vi "SearchTemplates.vi"(10 "Search Text":string, 11 "Filtered Templates":refnum<class "MetaDataObj.lvclass">[](array[class])) -> (3 "Display Templates":refnum<class "MetaDataObj.lvclass">[](array[class]))   [LabVIEW 2016]
uses:
  <resource>/dialog/NewProjectWizard/MetaDataObj/MetaDataObj.lvclass
  <resource>/dialog/NewProjectWizard/MetaDataObj/Accessors/Read Title.vi
  <resource>/dialog/NewProjectWizard/MetaDataObj/Accessors/Read Keywords.vi
  <resource>/dialog/NewProjectWizard/MetaDataObj/Accessors/Read Description.vi
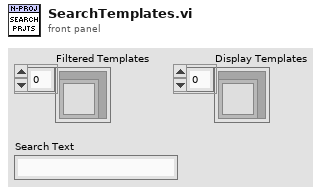
[diagram p1: front panel]
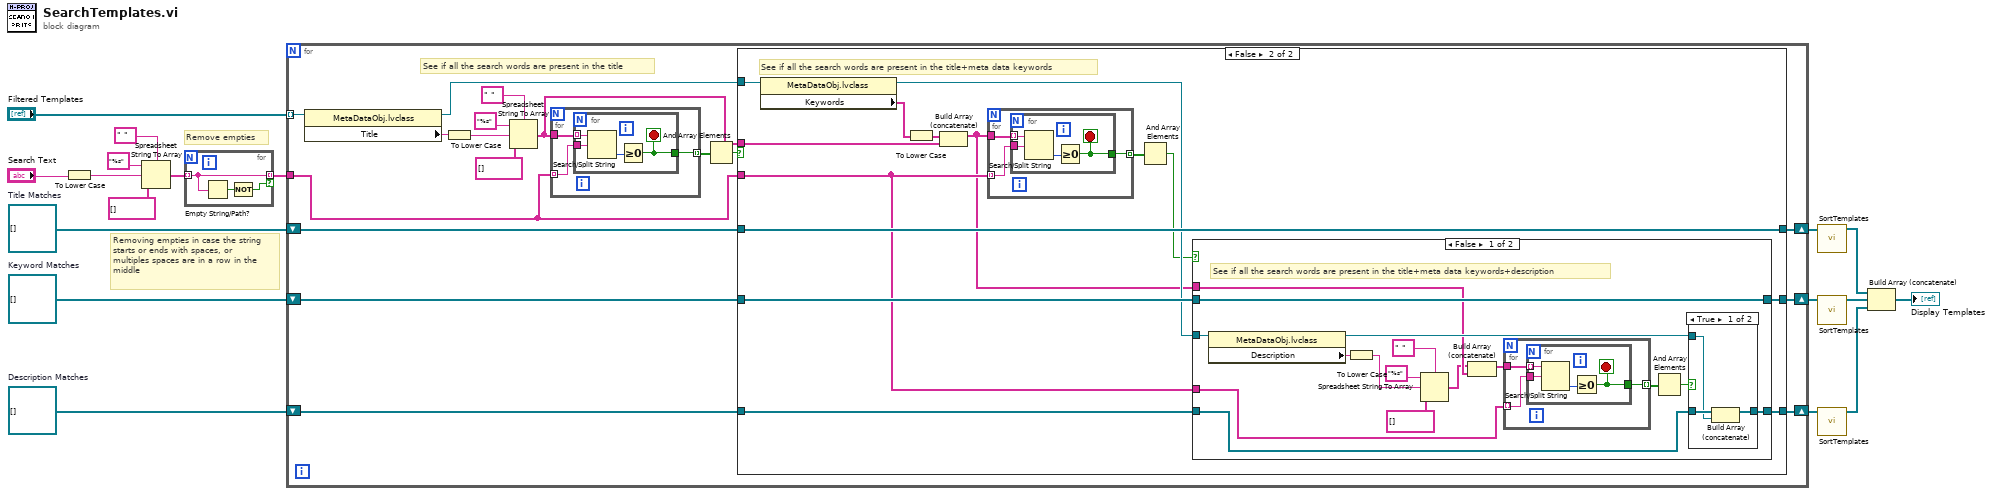
[diagram p0: block diagram]
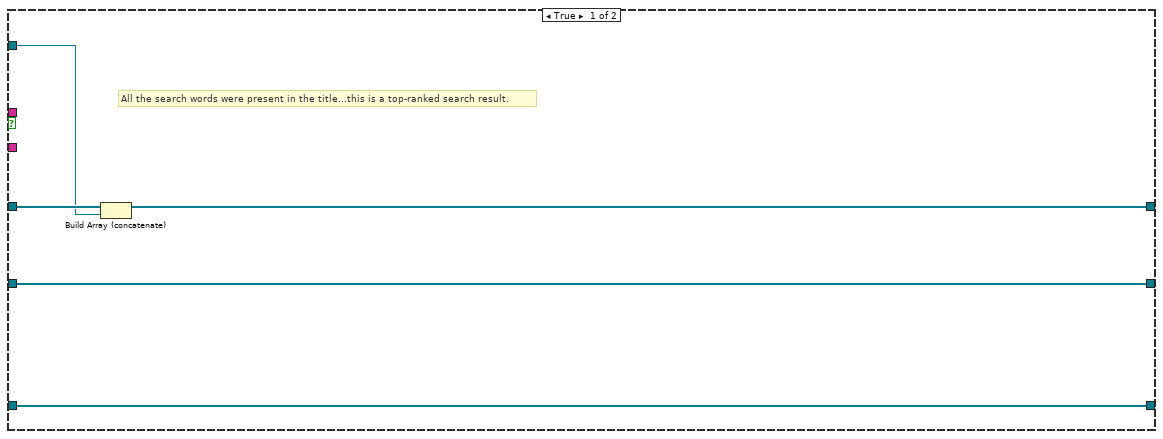
[diagram p2: hidden frame]
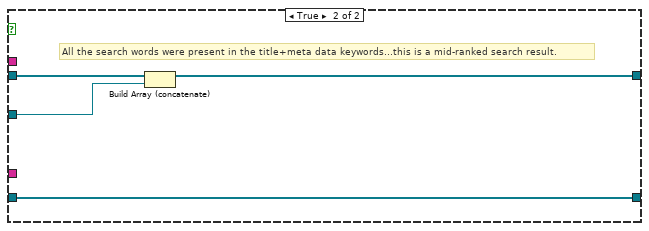
[diagram p4: hidden frame]
diagram:
  w15 = refnum<class "MetaDataObj.lvclass">[] []  # Description Matches
  w16 = refnum<class "MetaDataObj.lvclass">[] []  # Keyword Matches
  w17 = refnum<class "MetaDataObj.lvclass">[] []  # Title Matches
  # "Removing empties in case the string starts or ends with spaces, or multiples spaces are in a row in the middle"
  # "Remove empties"
  n1 = To Lower Case(string="Search Text") -> (all lower case string=w6:string)
  n2 = Spreadsheet String To Array(delimiter (Tab)=" ", format string="%s", spreadsheet string=w6, array type (2D Dbl)=string[] []) -> (array=w2:string[])
  n3 = for {
    tunnel: w2 -> [w21] mode=indexing
    tunnel: [w21] -> w1 mode=indexing if=w19
    n4 = Empty String/Path?(string/path=w21) -> (empty?=w20:bool)
    n5 = Not(x=w20) -> (.not. x?=w19:bool)
  }
  n6 = for {
    tunnel: "Filtered Templates" -> [w38] mode=indexing
    tunnel: w1 -> [w24]
    shift-right: [w34] -> w12
    shift-left: w17 -> [w37]
    shift-right: [w33] -> w13
    shift-left: w16 -> [w36]
    shift-right: [w32] -> w14
    shift-left: w15 -> [w35]
    # "See if all the search words are present in the title"
    n7 = property class="MetaDataObj.lvclass"(reference=w38) -> (reference out=w29:refnum<class "MetaDataObj.lvclass">, "Title"=w31:string)  [unwired: 1 in, 1 out]
    n8 = To Lower Case(string=w31) -> (all lower case string=w25:string)
    n9 = Spreadsheet String To Array(delimiter (Tab)=" ", format string="%s", spreadsheet string=w25, array type (2D Dbl)=string[] []) -> (array=w22:string[])
    n10 = for {
      tunnel: w22 -> [w39]
      tunnel: w24 -> [w41] mode=indexing
      tunnel: [w40] -> w23 mode=indexing
      n11 = for {
        tunnel: w41 -> [w45]
        tunnel: [w43] -> w40
        tunnel: w39 -> [w42] mode=indexing
        stop <- w43 stop-if-true
        n12 = Search/Split String(string=w42, search string/char (-)=w45) -> (offset of match=w44:i32)  [unwired: 1 in, 2 out]
        n13 = Greater Or Equal To 0?(x=w44) -> (x >= 0?=w43:bool)
      }
    }
    n14 = And Array Elements(Boolean array=w23) -> (logical AND=w30:bool)
    n15 = case shown="False" w30 {
      tunnel: w29 -> [w49 w64]
      tunnel: w37 -> [w50 w63]
      tunnel: w36 -> [w47 w62]
      tunnel: w35 -> [w46 w61]
      tunnel: [w48 w63] -> w34
      tunnel: [w47 w60] -> w33
      tunnel: [w46 w59] -> w32
      tunnel: w24 -> [_ w56]
      tunnel: w22 -> [_ w52]
      frame True {
        # "All the search words were present in the title...this is a top-ranked search result."
        n16 = Build Array (concatenate)(w50, w49) -> (w48:refnum<class "MetaDataObj.lvclass">[])
      }
      frame False {
        # "See if all the search words are present in the title+meta data keywords"
        n17 = property class="MetaDataObj.lvclass"(reference=w64) -> (reference out=w58:refnum<class "MetaDataObj.lvclass">, "Keywords"=w57:string[])  [unwired: 1 in, 1 out]
        n18 = To Lower Case(string=w57) -> (all lower case string=w55:string[])
        n19 = Build Array (concatenate)(w55, w52) -> (w51:string[])
        n20 = for {
          tunnel: w51 -> [w66]
          tunnel: w56 -> [w67] mode=indexing
          tunnel: [w65] -> w54 mode=indexing
          n21 = for {
            tunnel: w66 -> [w71] mode=indexing
            tunnel: w67 -> [w70]
            tunnel: [w68] -> w65
            stop <- w68 stop-if-true
            n22 = Search/Split String(string=w71, search string/char (-)=w70) -> (offset of match=w69:i32)  [unwired: 1 in, 2 out]
            n23 = Greater Or Equal To 0?(x=w69) -> (x >= 0?=w68:bool)
          }
        }
        n24 = And Array Elements(Boolean array=w54) -> (logical AND=w53:bool)
        n25 = case shown="False" w53 {
          tunnel: w62 -> [w87 w102]
          tunnel: w61 -> [w81 w99]
          tunnel: [w87 w100] -> w60
          tunnel: w58 -> [w86 w101]
          tunnel: [w85 w99] -> w59
          tunnel: w56 -> [w77 _]
          tunnel: w51 -> [w78 _]
          frame False {
            # "See if all the search words are present in the title+meta data keywords+description"
            n26 = property class="MetaDataObj.lvclass"(reference=w86) -> (reference out=w84:refnum<class "MetaDataObj.lvclass">, "Description"=w83:string)  [unwired: 1 in, 1 out]
            n27 = To Lower Case(string=w83) -> (all lower case string=w73:string)
            n28 = Spreadsheet String To Array(delimiter (Tab)=" ", format string="%s", spreadsheet string=w73, array type (2D Dbl)=string[] []) -> (array=w72:string[])
            n29 = Build Array (concatenate)(w72, w78) -> (w79:string[])
            n30 = for {
              tunnel: w79 -> [w89]
              tunnel: w77 -> [w90] mode=indexing
              tunnel: [w88] -> w80 mode=indexing
              n31 = for {
                tunnel: w89 -> [w94] mode=indexing
                tunnel: w90 -> [w93]
                tunnel: [w91] -> w88
                stop <- w91 stop-if-true
                n32 = Search/Split String(string=w94, search string/char (-)=w93) -> (offset of match=w92:i32)  [unwired: 1 in, 2 out]
                n33 = Greater Or Equal To 0?(x=w92) -> (x >= 0?=w91:bool)
              }
            }
            n34 = And Array Elements(Boolean array=w80) -> (logical AND=w82:bool)
            n35 = case shown="True" w82 {
              tunnel: w81 -> [w97 w98]
              tunnel: [w95 w98] -> w85
              tunnel: w84 -> [w96 _]
              frame True {
                n36 = Build Array (concatenate)(w97, w96) -> (w95:refnum<class "MetaDataObj.lvclass">[])
              }
              frame False {
              }
            }
          }
          frame True {
            # "All the search words were present in the title+meta data keywords...this is a mid-ranked search result."
            n37 = Build Array (concatenate)(w102, w101) -> (w100:refnum<class "MetaDataObj.lvclass">[])
          }
        }
      }
    }
  }
  n38 = call <resource>:"SortTemplates.vi"("Unsorted Templates"=w12) -> ("Sorted Templates"=w11:refnum<class "MetaDataObj.lvclass">[])  [unwired: 10 in]
  n39 = call <resource>:"SortTemplates.vi"("Unsorted Templates"=w13) -> ("Sorted Templates"=w10:refnum<class "MetaDataObj.lvclass">[])  [unwired: 10 in]
  n40 = call <resource>:"SortTemplates.vi"("Unsorted Templates"=w14) -> ("Sorted Templates"=w9:refnum<class "MetaDataObj.lvclass">[])  [unwired: 10 in]
  n41 = Build Array (concatenate)(w11, w10, w9) -> (→"Display Templates":refnum<class "MetaDataObj.lvclass">[])
